vi "KISSIA_TO ARRAY_REPETICIONES.vi"(10 "String":string="Numero de repeticiones: 5") -> (1 "Array":string[](array[string]))   [LabVIEW 2017]
panel:
  # "Numero de repeticiones: 5"
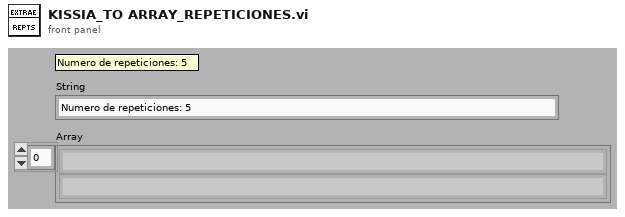
[diagram p1: front panel]
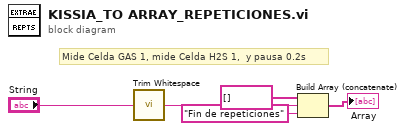
[diagram p0: block diagram]
diagram:
  # "Mide Celda GAS 1, mide Celda H2S 1,  y pausa 0.2s"
  n1 = call <vilib>:"Trim Whitespace.vi"("string"="String") -> ("trimmed string"=w2:string)  [unwired: 1 in]
  n2 = Build Array (concatenate)(string[] [] ("Array I"), w2, "Fin de repeticiones" ("element")) -> (→"Array":string[])
